vi "Servo_GP_Angle_Conversion_R0.vi"(8 "GP in":u16, 9 "Angle In":sgl, 10 "Mode Select":i32, 11 "Mount Offset":dbl=45.0 format="%#_13g") -> (1 "Angle Out":sgl, 2 "GP out":u16)   [LabVIEW 2015]
panel:
  # "0 = GP to Angle\n1 = Angle to GP"
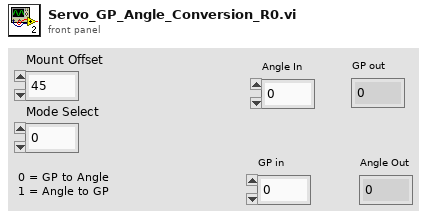
[diagram p1: front panel]
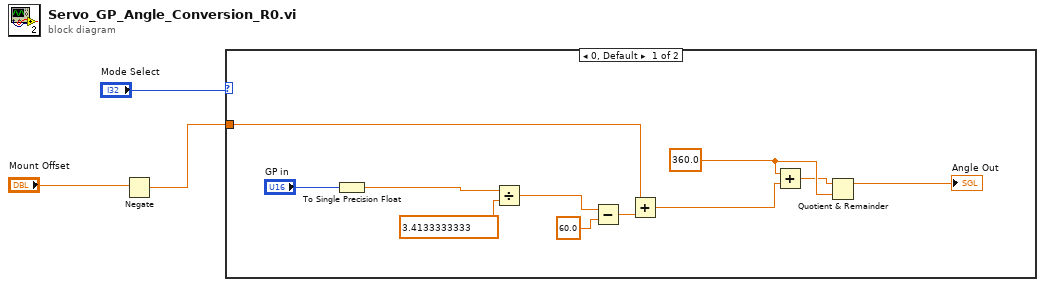
[diagram p0: block diagram]
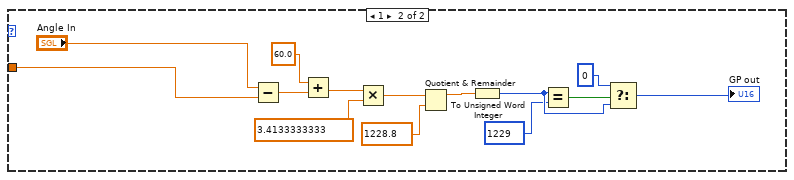
[diagram p2: hidden frame]
diagram:
  n1 = Negate(x="Mount Offset") -> (-x=w1:dbl)
  n2 = case shown="0, Default" "Mode Select" {
    tunnel: w1 -> [w4 w15]
    frame 0, Default {
      w13 = 360.0
      n3 = To Single Precision Float(number="GP in") -> (single precision float=w5:sgl)
      n4 = Divide(x=w5, y=3.4133333333) -> (x/y=w8:dbl)
      n5 = Subtract(x=w8, y=60.0) -> (x-y=w10:dbl)
      n6 = Add(x=w4, y=w10) -> (x+y=w11:dbl)
      n7 = Add(x=w13, y=w11) -> (x+y=w12:dbl)
      n8 = Quotient & Remainder(x=w12, y=w13) -> (x-y*floor(x/y)=→"Angle Out":dbl)  [unwired: 1 out]
    }
    frame 1 {
      n9 = Subtract(x="Angle In", y=w15) -> (x-y=w27:dbl)
      n10 = Add(x=60.0, y=w27) -> (x+y=w25:dbl)
      n11 = Multiply(x=w25, y=3.4133333333) -> (x*y=w23:dbl)
      n12 = Quotient & Remainder(x=w23, y=1228.8) -> (x-y*floor(x/y)=w19:dbl)  [unwired: 1 out]
      n13 = To Unsigned Word Integer(number=w19) -> (unsigned 16bit integer=w18:u16)
      n14 = Equal?(x=w18, y=u16 1229) -> (x = y?=w22:bool)
      n15 = Select(t=u16 0, s=w22, f=w18) -> (s? t:f=→"GP out":u16)
    }
  }
